vi "Effective Rate Percent.vi"(8 "error in (no error)":errorcluster, 10 "Set Rate (Percent) in":dbl, 11 "Elevator in":refnum<class "Elevator.lvclass">) -> (0 "error out":errorcluster, 2 "Set Rate (Percent) out":dbl, 3 "Elevator out":refnum<class "Elevator.lvclass">)   [LabVIEW 2014, in "Elevator.lvlib" / "Elevator.lvclass"]
uses:
  Elevator.lvclass
  Elevator.lvclass/Elevator.ctl
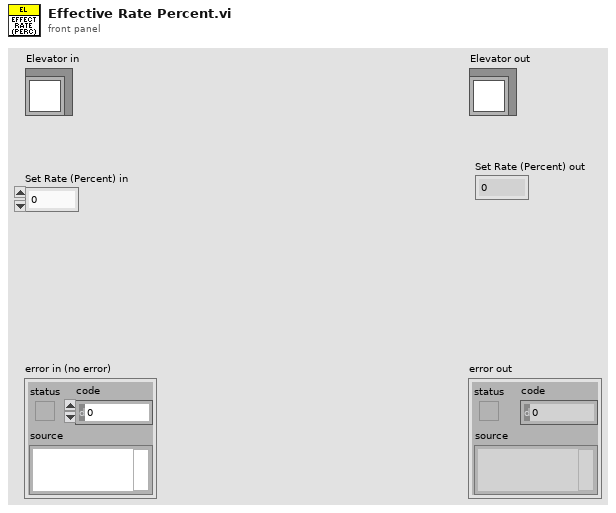
[diagram p1: front panel]
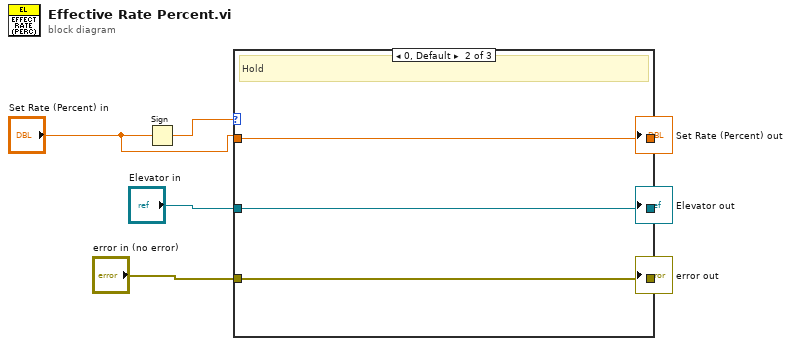
[diagram p0: block diagram]
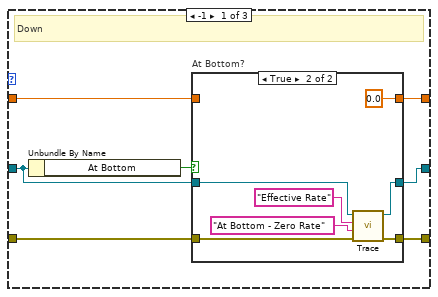
[diagram p2: hidden frame]
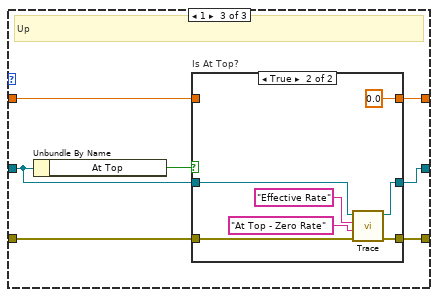
[diagram p4: hidden frame]
diagram:
  n1 = Sign(1:"Set Rate (Percent) in") -> (0:w4:dbl)
  n2 = case shown="0, Default" w4 {
    tunnel: "Elevator in" -> [w9 w26 w31]
    tunnel: [w8 w26 w30] -> w6
    tunnel: [w13 w27 w33] -> w5
    tunnel: "Set Rate (Percent) in" -> [w12 w27 w32]
    tunnel: "error in (no error)" -> [w11 w25 w29]
    tunnel: [w10 w25 w28] -> w2
    frame -1 {
      # "Down"
      n3 = Unbundle By Name(w9) -> ("At Bottom"=w14:bool)
      n4 = case "At Bottom?" shown="True" w14 {
        tunnel: [w17 0.0] -> w13
        tunnel: w12 -> [w17 _]
        tunnel: w11 -> [w16 w23]
        tunnel: [w16 w22] -> w10
        tunnel: w9 -> [w15 w21]
        tunnel: [w15 w20] -> w8
        frame False {
        }
        frame True {
          n5 = call-dynamic "Trace.vi"("error in (no error)"=w23, "System Message"="At Bottom - Zero Rate", "System Action"="Effective Rate", "System Actor in"=w21) -> ("error out"=w22:errorcluster, "System Actor out"=w20:refnum<class "Elevator.lvclass">)  [unwired: 6 in]
        }
      }
    }
    frame 0, Default {
      # "Hold"
    }
    frame 1 {
      # "Up"
      n6 = Unbundle By Name(w31) -> ("At Top"=w34:bool)
      n7 = case "Is At Top?" shown="True" w34 {
        tunnel: [w37 0.0] -> w33
        tunnel: w32 -> [w37 _]
        tunnel: w31 -> [w36 w43]
        tunnel: [w36 w42] -> w30
        tunnel: w29 -> [w35 w39]
        tunnel: [w35 w38] -> w28
        frame False {
        }
        frame True {
          n8 = call-dynamic "Trace.vi"("error in (no error)"=w39, "System Message"="At Top - Zero Rate", "System Action"="Effective Rate", "System Actor in"=w43) -> ("error out"=w38:errorcluster, "System Actor out"=w42:refnum<class "Elevator.lvclass">)  [unwired: 6 in]
        }
      }
    }
  }
  "error out" <- w2
  "Elevator out" <- w6
  "Set Rate (Percent) out" <- w5
